vi "NanonisProperties_nano.vi"(0 "Application reference":refnum<vi>, 1 "Z Write (m)":sgl format="%#_6p", 5 "X pen (nm)":dbl, 7 "Z pen (nm)":dbl, 11 "Error in":errorcluster, 12 "Z Write?":bool) -> (2 "Frame Size (m)":cluster{"Width":sgl, "Height":sgl} {"Height" format="%.2p"; "Width" format="%.2p"}, 3 "Frame Origin (m)":cluster{"Xc":sgl, "Yc":sgl} {"Yc" format="%.2p"; "Xc" format="%.2p"}, 4 "Application ref out":refnum<vi>, 6 "Setpoint (A)":sgl format="%#_6p", 8 "Current (pA)":sgl format="%#_6p", 10 "Z Read (m)":sgl format="%#_6p", 15 "error out":errorcluster)   [LabVIEW 2017]
uses:
  Program Files/National Instruments/LabVIEW 2019/user.lib/Nanonis Prog Interface V5/Nanonis Prog Interface.lvlib
panel:
  out "prog int?":bool
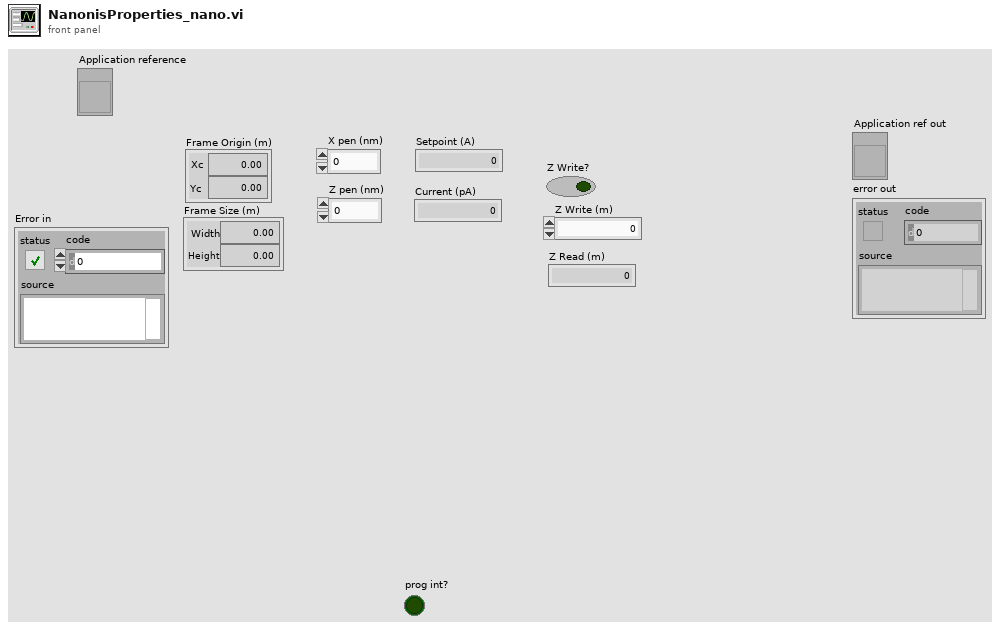
[diagram p1: front panel]
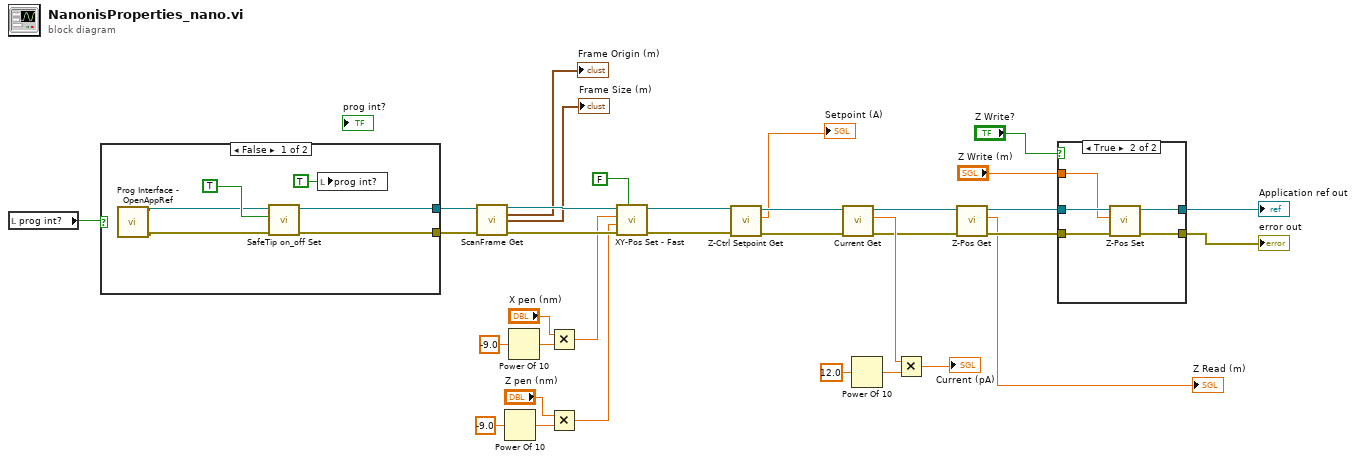
[diagram p0: block diagram]
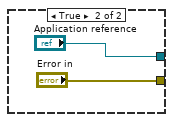
[diagram p3: hidden frame]
diagram:
  n1 = local read "prog int?"() -> (w3:bool)
  n2 = case shown="False" w3 {
    tunnel: [w38 "Application reference"] -> w33
    tunnel: [w37 "Error in"] -> w32
    frame False {
      n3 = call <userlib>:"Prog Interface - OpenAppRef.vi"() -> ("Error out"=w35:errorcluster, "Application reference"=w36:refnum<vi>)  [unwired: 6 in]
      n4 = call <userlib>:"SafeTip on_off Set.vi"("error in (no error)"=w35, "SafeTip ON/OFF"=TRUE, "Application ref in"=w36) -> ("error out"=w37:errorcluster, "Application ref out"=w38:refnum<vi>)  [unwired: 7 in]
      n5 = local write "prog int?"(TRUE ("prog int?")) -> ()
    }
    frame True {
    }
  }
  n6 = call <userlib>:"ScanFrame Get.vi"("Application ref in"=w33, "error in (no error)"=w32) -> ("Application ref out"=w31:refnum<vi>, "Center coordinates (m)"=→"Frame Origin (m)":cluster{"Xc":sgl, "Yc":sgl}, "Size (m)"=→"Frame Size (m)":cluster{"Width":sgl, "Height":sgl}, "error out"=w30:errorcluster)  [unwired: 9 in, 1 out]
  n7 = Power Of 10(x=-9.0) -> (10^x=w24:dbl)
  n8 = Power Of 10(x=-9.0) -> (10^x=w27:dbl)
  n9 = Multiply(x="X pen (nm)", y=w27) -> (x*y=w21:dbl)
  n10 = Multiply(x="Z pen (nm)", y=w24) -> (x*y=w20:dbl)
  n11 = call <userlib>:"XY-Pos Set - Fast.vi"("Wait end-of-motion (T=True)"=FALSE, "error in (no error)"=w30, "Y (m)"=w20, "X (m)"=w21, "Application ref in"=w31) -> ("error out"=w14:errorcluster, "Application ref out"=w15:refnum<vi>)  [unwired: 4 in]
  n12 = call <userlib>:"Z-Ctrl Setpoint Get.vi"("error in (no error)"=w14, "Application ref in"=w15) -> ("error out"=w12:errorcluster, "Z Controller setpoint"=→"Setpoint (A)":sgl, "Application ref out"=w13:refnum<vi>)  [unwired: 6 in]
  n13 = call <userlib>:"Current Get.vi"("Error in (no error)"=w12, "Application ref in"=w13) -> ("Error out"=w10:errorcluster, "Current (A)"=w16:sgl, "Application ref out"=w11:refnum<vi>)  [unwired: 5 in]
  n14 = Power Of 10(x=12.0) -> (10^x=w17:dbl)
  n15 = Multiply(x=w16, y=w17) -> (x*y=→"Current (pA)":dbl)
  n16 = call <userlib>:"Z-Pos Get.vi"("error in (no error)"=w10, "Application ref in"=w11) -> ("error out"=w8:errorcluster, "Z position (m)"=→"Z Read (m)":sgl, "Application ref out"=w9:refnum<vi>)  [unwired: 7 in]
  n17 = case shown="True" "Z Write?" {
    tunnel: w9 -> [w44 w49]
    tunnel: w8 -> [w43 w48]
    tunnel: [w44 w47] -> w7
    tunnel: [w43 w46] -> w6
    tunnel: "Z Write (m)" -> [_ w45]
    frame False {
    }
    frame True {
      n18 = call <userlib>:"Z-Pos Set.vi"("error in (no error)"=w48, "Z position (m)"=w45, "Application ref in"=w49) -> ("error out"=w46:errorcluster, "Application ref out"=w47:refnum<vi>)  [unwired: 7 in]
    }
  }
  "Application ref out" <- w7
  "error out" <- w6
